vi "Switch_GetAllInstrumentNames.vi"(8 "error in (no error)":errorcluster, 11 "Semiconductor Module Context":T1) -> (0 "error out":errorcluster, 1 "Channel Lists":string[](array[string]), 2 "Instrument Names":string[](array[string]), 3 "Semiconductor Module Context Out":T1)   [LabVIEW 2014]
uses:
  <vilib>/NI_TestStand_SemiconductorModule/NI_TestStand_Semiconductor_Module.lvlibp/PinMap/General/SemiconductorModuleContext.ctl
  <vilib>/NI_TestStand_SemiconductorModule/NI_TestStand_Semiconductor_Module.lvlibp
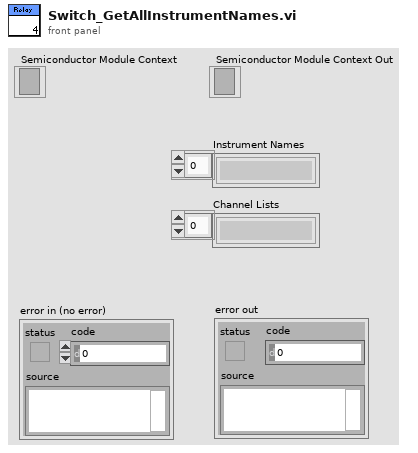
[diagram p1: front panel]
types:
  T1 = typedef "NI_TestStand_Semiconductor_Module.lvlibp/SemiconductorModuleContext.ctl" = refnum<k7>
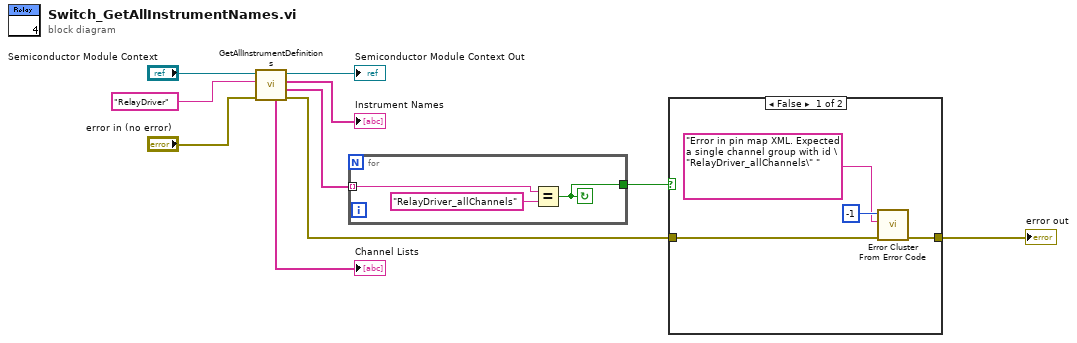
[diagram p0: block diagram]
diagram:
  n1 = call <vilib>:"GetAllInstrumentDefinitions.vi"("error in (no error)"="error in (no error)", "Instrument Type Id"="RelayDriver" ("Instrument Type"), "Semiconductor Module Context"="Semiconductor Module Context") -> ("error out"=w4:errorcluster, "Channel Group Ids"=w3:string[], "Instrument Names"=→"Instrument Names":string[], "Semiconductor Module Context Out"=→"Semiconductor Module Context Out":T1, "Channel Lists"=→"Channel Lists":string[])  [unwired: 4 in]
  n2 = for {
    tunnel: w3 -> [w13] mode=indexing
    tunnel: [w11] -> w10
    stop <- w11 continue-if-true
    n3 = Equal?(x=w13, y="RelayDriver_allChannels" ("delimiter (Tab)")) -> (x = y?=w11:bool)
  }
  n4 = case shown="False" w10 {
    tunnel: w4 -> [w14 w18]
    tunnel: [w17 w18] -> w9
    frame False {
      n5 = call <vilib>:"Error Cluster From Error Code.vi"("error in (no error)"=w14, "error message (\"\")"="Error in pin map XML. Expected a single channel group with id \"RelayDriver_allChannels\" " ("source"), "error code (0)"=-1 ("code")) -> ("error out"=w17:errorcluster)  [unwired: 6 in]
    }
    frame True {
    }
  }
  "error out" <- w9
